vi "Read Z_State.vi"(11 "HE1_Z_state in":refnum<class "HE_Z_state.lvclass">) -> (2 "Z_State_heating":T1=enum."on min", 3 "HE1_Z_state out":refnum<class "HE_Z_state.lvclass">)   [LabVIEW 2019, in "Heating.lvlib" / "HE_Z_state.lvclass"]
uses:
  HE_Z_state.lvclass
  ctl/Z_State.ctl
  HE_Z_state.lvclass/HE_Z_state.ctl
  Heating.lvlib
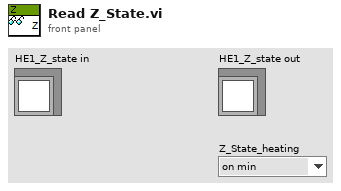
[diagram p1: front panel]
types:
  T1 = typedef "Heating.lvlib/Z_State.ctl" = enum8{"initialization", "alarm", "disabled", "not ready", "stop ready", "reserv", "switched off", "reserv2", "switched on", "check", "on min", "decrease out", "on", "increase out", "on max"}
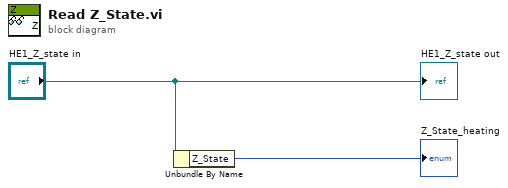
[diagram p0: block diagram]
diagram:
  n1 = Unbundle By Name("HE1_Z_state in") -> ("Z_State"=→"Z_State_heating":T1)
  "HE1_Z_state out" <- "HE1_Z_state in"
